vi "Main.vi"() -> ()   [LabVIEW 2017, in "Graveyard.lvlib"]
uses:
  Graveyard.lvlib
  Private/Bookmarks Type.ctl
  Private/State.ctl
panel:
  in  "Bookmarks Type":T1
  in  "Help":bool
  in  "Close":bool
  in  "Graves":string(tree)
  in  "Scope":u16(ring) items=["Main Application Instance", "Eulogy.lvproj"]
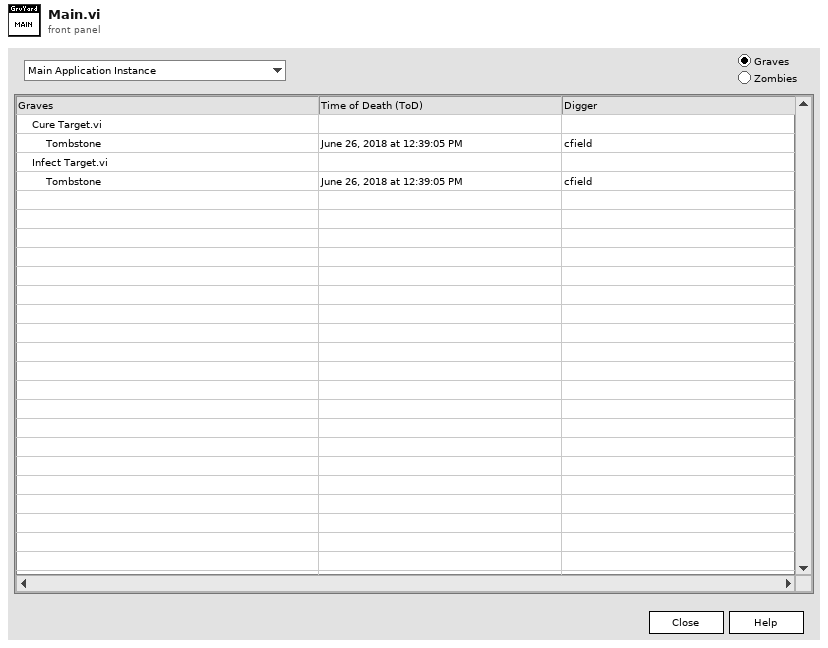
[diagram p1: front panel]
types:
  T1 = typedef "Graveyard.lvlib/Bookmarks Type.ctl" = enum32{"Graves", "Zombies"}
  T2 = typedef "Graveyard.lvlib/State.ctl" = cluster{"Bookmarks":refnum<vi>, "Bookmarks Type":T1, "Front Panel":refnum<vi>, "Scopes":refnum<vi>}
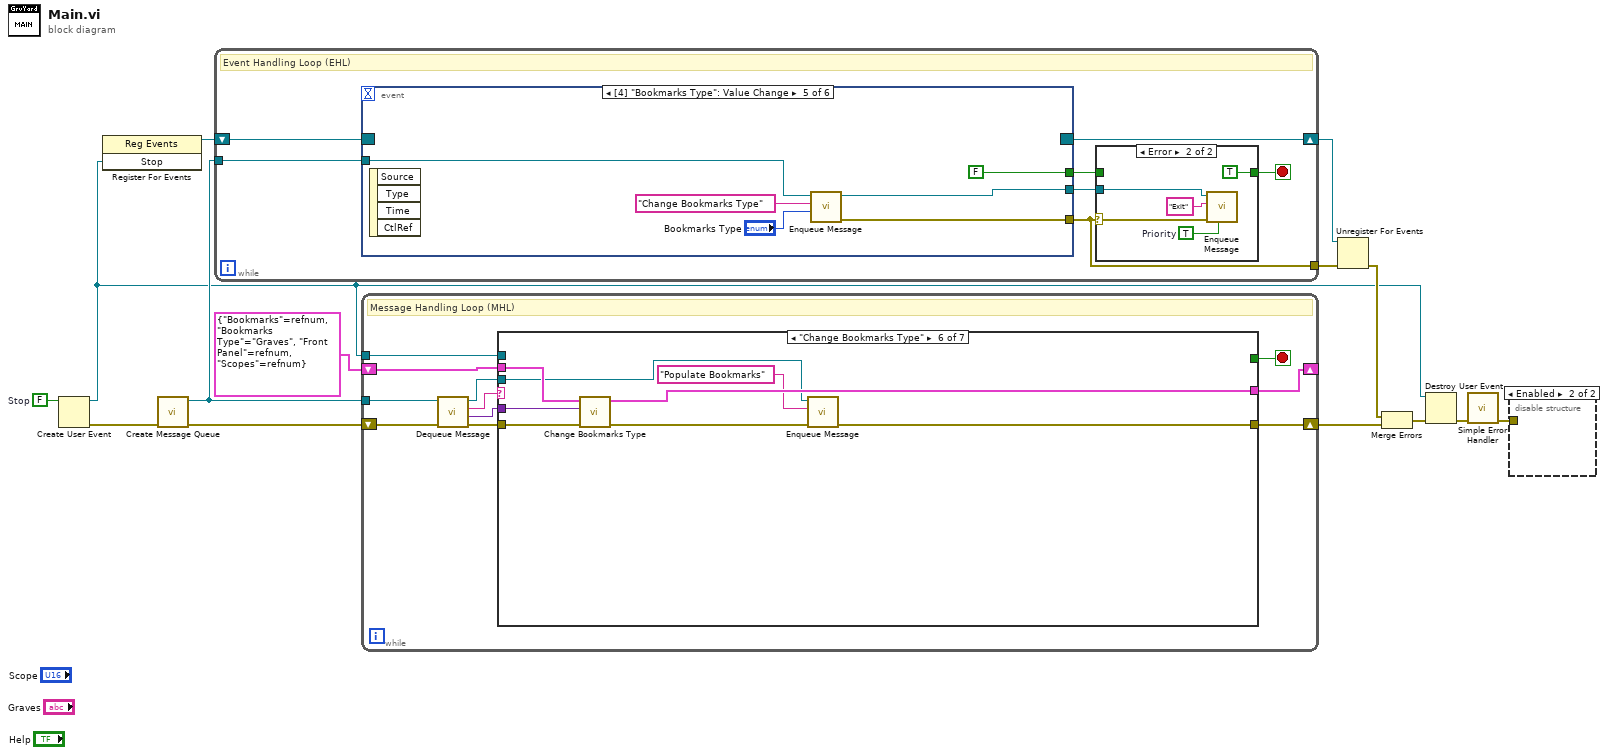
[diagram p0: block diagram]
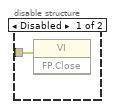
[diagram p2: hidden frame]
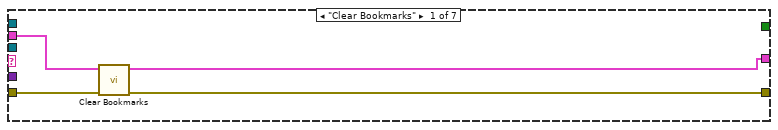
[diagram p3: hidden frame]
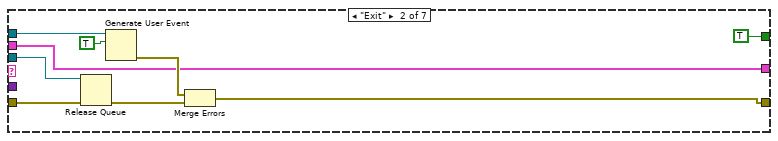
[diagram p4: hidden frame]
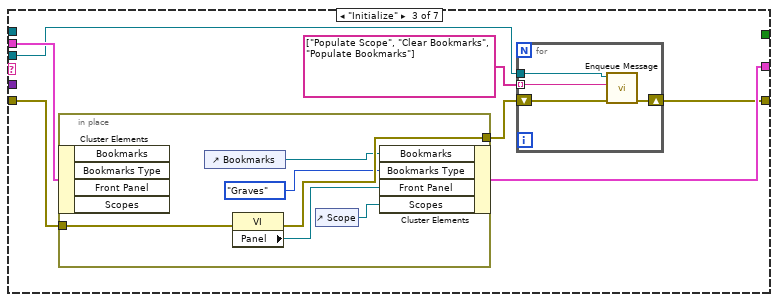
[diagram p5: hidden frame]
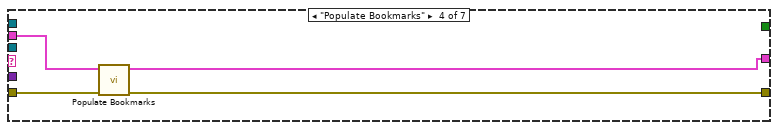
[diagram p6: hidden frame]
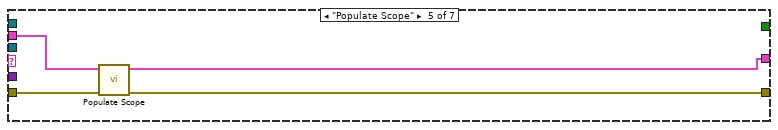
[diagram p7: hidden frame]
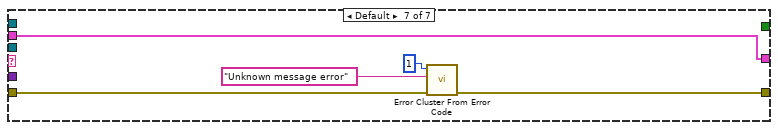
[diagram p8: hidden frame]
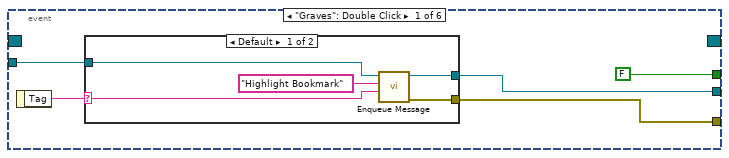
[diagram p10: hidden frame]
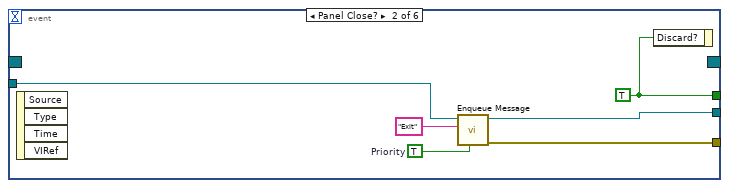
[diagram p12: hidden frame]
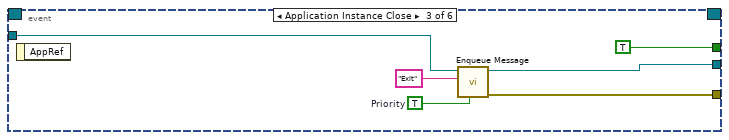
[diagram p13: hidden frame]
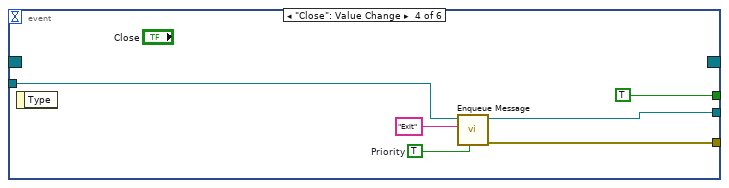
[diagram p14: hidden frame]
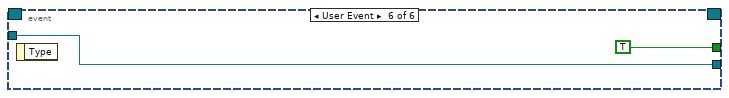
[diagram p15: hidden frame]
diagram:
  w11 = FALSE  # Stop
  n1 = Create User Event(user event datatype=w11) -> (user event=w4:refnum<user-event>, error out=w10:errorcluster)  [unwired: 1 in]
  n2 = register-events(w4) -> (reference out=w14:refnum<event-registration>)  [unwired: 2 in, 1 out]
  n3 = call "Create Message Queue.vi"("Error In"=w10) -> ("Error Out"=w8:errorcluster, "Message Queue"=w9:refnum<queue>)  [unwired: 9 in]
  n4 = while {
    shift-right: [w20] -> w13
    shift-left: w14 -> [w21]
    tunnel: [w17] -> w12
    tunnel: w9 -> [w15]
    stop <- w18 stop-if-true
    # "Event Handling Loop (EHL)"
    n5 = event shown="[4] \"Bookmarks Type\": Value Change" {
      selector: w21 -> [_ _ _ _ _ _]
      dyn-events: [_ _ _ _ _ _] -> w20
      timeout: _ -> [_ _ _ _ _ _]
      tunnel: [w32 w42 w49 w55 w61 _] -> w17
      tunnel: [FALSE w44 TRUE TRUE FALSE TRUE] -> w19
      tunnel: [w30 w43 w50 w56 w62 w64] -> w16
      tunnel: w15 -> [w28 w39 w46 w52 w59 w64]
      event "Graves": Double Click {
        n6 = event-data() -> ("Tag"=w29:string)  [unwired: 1 in]
        n7 = case shown="Default" w29 {
          selector: w29 -> [w34 _]
          tunnel: [w36 _] -> w32
          tunnel: [w37 w38] -> w30
          tunnel: w28 -> [w33 w38]
          frame Default {
            n8 = call "Enqueue Message.vi"("Data"=w34, "Command"="Highlight Bookmark", "Message Queue In"=w33) -> ("Error Out"=w36:errorcluster, "Message Queue Out"=w37:refnum<queue>)  [unwired: 7 in]
          }
          frame "" {
          }
        }
      }
      event Panel Close? {
        w40 = TRUE  # Priority
        w44 = TRUE
        n9 = event-data() -> ()  [unwired: 1 in, 4 out]
        n10 = call "Enqueue Message.vi"("Priority"=w40, "Command"="Exit", "Message Queue In"=w39) -> ("Error Out"=w42:errorcluster, "Message Queue Out"=w43:refnum<queue>)  [unwired: 7 in]
        n11 = event-data("Discard?"=w44) -> ()  [unwired: 1 in, 1 out]
      }
      event Application Instance Close {
        w47 = TRUE  # Priority
        n12 = event-data() -> ()  [unwired: 1 in, 1 out]
        n13 = call "Enqueue Message.vi"("Priority"=w47, "Command"="Exit", "Message Queue In"=w46) -> ("Error Out"=w49:errorcluster, "Message Queue Out"=w50:refnum<queue>)  [unwired: 7 in]
      }
      event "Close": Value Change {
        w53 = TRUE  # Priority
        n14 = event-data() -> ()  [unwired: 1 in, 1 out]
        n15 = call "Enqueue Message.vi"("Priority"=w53, "Command"="Exit", "Message Queue In"=w52) -> ("Error Out"=w55:errorcluster, "Message Queue Out"=w56:refnum<queue>)  [unwired: 7 in]
      }
      event Value Change {
        n16 = event-data() -> ()  [unwired: 1 in, 4 out]
        n17 = call "Enqueue Message.vi"("Data"="Bookmarks Type", "Command"="Change Bookmarks Type", "Message Queue In"=w59) -> ("Error Out"=w61:errorcluster, "Message Queue Out"=w62:refnum<queue>)  [unwired: 7 in]
      }
      event User Event {
        n18 = event-data() -> ()  [unwired: 1 in, 1 out]
      }
    }
    n19 = case shown="Error" w17 {
      selector: w17 -> [_ w27]
      tunnel: w19 -> [w22 _]
      tunnel: [w22 TRUE] -> w18
      tunnel: w16 -> [_ w25]
      frame No Error {
      }
      frame Error {
        w23 = TRUE  # Priority
        n20 = call "Enqueue Message.vi"("Priority"=w23, "Error In"=w27, "Command"="Exit", "Message Queue In"=w25) -> ()  [unwired: 6 in, 2 out]
      }
    }
  }
  n21 = while {
    tunnel: w9 -> [w75]
    shift-right: [w73] -> w6
    shift-left: w8 -> [w72]
    tunnel: w4 -> [w69]
    shift-right: [w66] -> _
    shift-left: T2 {"Bookmarks"=refnum, "Bookmarks Type"=enum."Graves", "Front Panel"=refnum, "Scopes"=refnum} ("State") -> [w67]
    stop <- w70 stop-if-true
    # "Message Handling Loop (MHL)"
    n22 = call "Dequeue Message.vi"("Error In"=w72, "Message Queue In"=w75) -> ("Error Out"=w71:errorcluster, "Data"=w65:variant, "Command"=w74:string, "Message Queue Out"=w68:refnum<queue>)  [unwired: 6 in]
    n23 = case shown="\"Change Bookmarks Type\"" w74 {
      tunnel: [w76 w86 w92 w106 w110 w116 w122] -> w73
      tunnel: w71 -> [w77 w88 w91 w107 w111 w121 w124]
      tunnel: [_ TRUE _ _ _ _ _] -> w70
      tunnel: w69 -> [_ w85 _ _ _ _ _]
      tunnel: w68 -> [_ w81 w93 _ _ w115 _]
      tunnel: w67 -> [w79 w80 w95 w109 w113 w118 w123]
      tunnel: [w78 w80 w94 w108 w112 w117 w123] -> w66
      tunnel: w65 -> [_ _ _ _ _ w119 _]
      frame "Clear Bookmarks" {
        n24 = call "Clear Bookmarks.vi"("Error In"=w77, "State In"=w79) -> ("Error Out"=w76:errorcluster, "State Out"=w78:T2)  [unwired: 8 in]
      }
      frame "Exit" {
        n25 = Release Queue(queue=w81, error in (no error)=w88) -> (error out=w82:errorcluster)  [unwired: 1 in, 2 out]
        n26 = Generate User Event(user event=w85, event data cluster=TRUE ("event data")) -> (error out=w83:errorcluster)  [unwired: 2 in, 1 out]
        n27 = Merge Errors(w83, w82) -> (w86:errorcluster)
      }
      frame "Initialize" {
        n28 = in-place {
          in-place-border: w91 -> [w105]
          in-place-border: [w104] -> w90
          n29 = in-place-cluster #1(w95) -> ()  [unwired: 4 out]
          n30 = control-ref of="Bookmarks"() -> (w103:refnum<vi>)
          n31 = property class="VI"(error in=w105) -> (error out=w104:errorcluster, "Panel"=w101:refnum<vi>)  [unwired: 1 in, 1 out]
          n32 = control-ref of="Scope"() -> (w102:refnum<vi>)
          n33 = in-place-cluster #1("Bookmarks"=w103, "Bookmarks Type"=Bookmarks_Type."Graves", "Front Panel"=w101, "Scopes"=w102) -> (w94:T2)
        }
        n34 = for {
          tunnel: w93 -> [w99]
          shift-right: [w98] -> w92
          shift-left: w90 -> [w97]
          tunnel: string[] ["Populate Scope", "Clear Bookmarks", "Populate Bookmarks"] -> [w96] mode=indexing
          n35 = call "Enqueue Message.vi"("Error In"=w97, "Command"=w96, "Message Queue In"=w99) -> ("Error Out"=w98:errorcluster)  [unwired: 7 in, 1 out]
        }
      }
      frame "Populate Bookmarks" {
        n36 = call "Populate Bookmarks.vi"("Error In"=w107, "State In"=w109) -> ("Error Out"=w106:errorcluster, "State Out"=w108:T2)  [unwired: 8 in]
      }
      frame "Populate Scope" {
        n37 = call "Populate Scope.vi"("Error In"=w111, "State In"=w113) -> ("Error Out"=w110:errorcluster, "State Out"=w112:T2)  [unwired: 8 in]
      }
      frame "Change Bookmarks Type" {
        n38 = call "Change Bookmarks Type.vi"("Error In"=w121, "Data"=w119, "State In"=w118) -> ("Error Out"=w120:errorcluster, "State Out"=w117:T2)  [unwired: 7 in]
        n39 = call "Enqueue Message.vi"("Error In"=w120, "Command"="Populate Bookmarks", "Message Queue In"=w115) -> ("Error Out"=w116:errorcluster)  [unwired: 7 in, 1 out]
      }
      frame Default {
        n40 = call <vilib>:"Error Cluster From Error Code.vi"("error in (no error)"=w124, "error message (\"\")"="Unknown message error" ("error message (\"\")"), "error code (0)"=1) -> ("error out"=w122:errorcluster)  [unwired: 6 in]
      }
    }
  }
  n41 = Unregister For Events(event registration refnum=w13, error in=w12) -> (error out=w7:errorcluster)
  n42 = Merge Errors(w7, w6) -> (w5:errorcluster)
  n43 = Destroy User Event(user event=w4, error in=w5) -> (error out=w3:errorcluster)
  n44 = call <vilib>:"Simple Error Handler.vi"("error in (no error)"=w3) -> ("error out"=w2:errorcluster)  [unwired: 4 in, 4 out]
  n45 = disable-structure shown="Enabled" {
    disable-tunnel: w2 -> [w127 _]
    frame Disabled {
      n46 = invoke class="VI" method="FP.Close"(error in=w127) -> ()  [unwired: 2 in, 3 out]
    }
    frame Enabled {
    }
  }
